vi "AgPSA _Poll PSA Freq Lock.vi"(8 "error in (no error)":errorcluster, 10 "Time Target (s)":dbl=15.0 format="%#_13g", 11 "VISA resource":refnum<visa-resource-name>="PSA1") -> (0 "error out":errorcluster, 3 "Locked":bool)   [LabVIEW 2015]
panel:
  out "Elapsed Time to Reference Lock":u32(slide) scale=0.0..15.0
  out "Elapsed Time (s)":u32 format="%<%H:%M:%S>t"
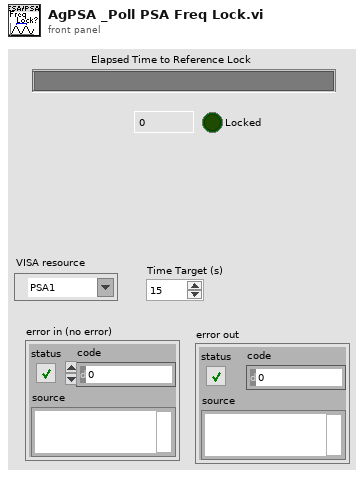
[diagram p1: front panel]
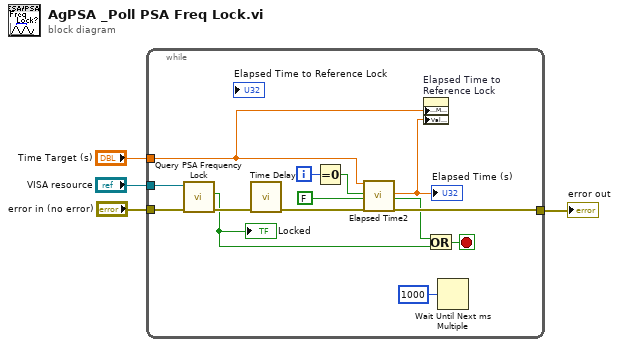
[diagram p0: block diagram]
diagram:
  n1 = while {
    tunnel: [w17] -> w1
    tunnel: "error in (no error)" -> [w10]
    tunnel: "VISA resource" -> [w9]
    tunnel: "Time Target (s)" -> [w7]
    i -> [w13]
    stop <- w14 stop-if-true
    n2 = call "Query PSA Frequency Lock.vi"("error in (no error)"=w10, "VISA resource"=w9) -> ("error out"=w16:errorcluster, "Locked"=w8:bool)  [unwired: 7 in, 1 out]
    "Locked" <- w8
    n3 = call "Time Delay"("error in (no error)"=w16) -> ("error out"=w18:errorcluster)  [unwired: 10 in]
    n4 = Equal To 0?(x=w13) -> (x = 0?=w12:bool)
    n5 = call "Elapsed Time2"("Time Target (s)"=w7, "Reset"=w12, "Auto Reset"=FALSE, "error in (no error)"=w18) -> ("Elapsed Time (s)"=w6:dbl, "Time has Elapsed"=w15:bool, "error out"=w17:errorcluster)  [unwired: 8 in, 5 out]
    "Elapsed Time (s)" <- w6
    n6 = property on="Elapsed Time to Reference Lock" class="Slide (strict)"("Scale.Maximum"=w7, "Value"=w6) -> ()  [unwired: 2 in, 2 out]
    n7 = Or(x=w15, y=w8) -> (x .or. y?=w14:bool)
    n8 = Wait Until Next ms Multiple(millisecond multiple=u32 1000) -> ()  [unwired: 1 out]
  }
  "error out" <- w1
